vi "example.vi"() -> ()   [LabVIEW 2019]
uses:
  d822b4ab-b711-45da-a8f1-ab7e2b244829.vi
  netCDFModule.py path constant.vi
panel:
  out "return value":dbl[][][][](array[numeric])
  in  "variable key":string
  in  "dimension key":string
  out "dimension":string
  in  "metadata key":string
  in  "file path":path
  out "error out":errorcluster
  out "metadata":string
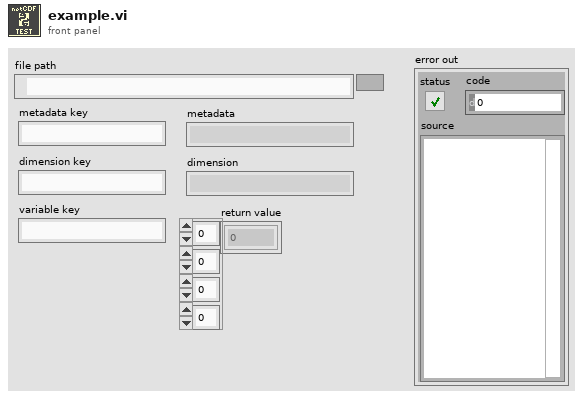
[diagram p1: front panel]
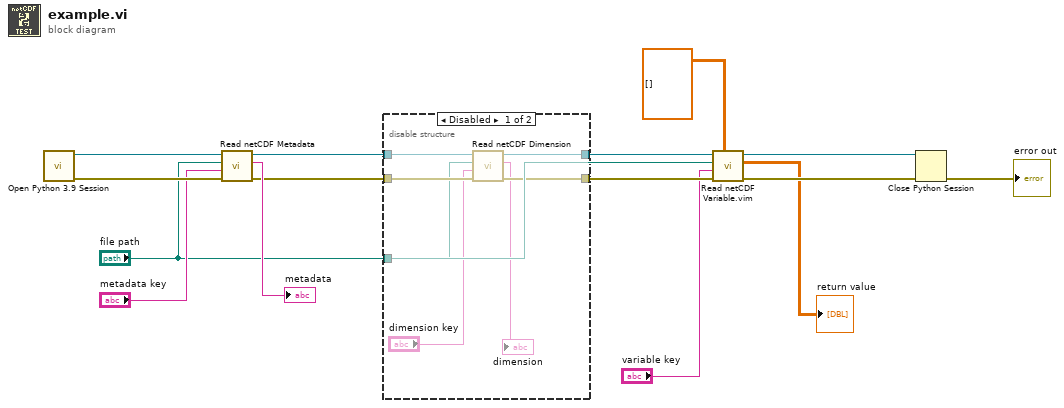
[diagram p0: block diagram]
diagram:
  n1 = call "Open Python 3.9 Session.vi"() -> ("error out"=w15:errorcluster, "Refnum out"=w12:refnum<k35>)  [unwired: 10 in]
  n2 = call "Read netCDF Metadata.vi"("error in (no error)"=w15, "key"="metadata key", "file path"="file path", "Refnum in"=w12) -> ("error out"=w9:errorcluster, "Value"=→"metadata":string, "Refnum out"=w10:refnum<k35>)  [unwired: 5 in]
  n3 = disable-structure shown="Disabled" {
    disable-tunnel: w10 -> [w22 w23]
    disable-tunnel: w9 -> [w21 w24]
    disable-tunnel: "file path" -> [w20 _]
    disable-tunnel: [w19 w23] -> w5
    disable-tunnel: [w18 w24] -> w4
    frame Disabled {
      n4 = call "Read netCDF Dimension.vi"("error in (no error)"=w21, "key"="dimension key", "file path"=w20, "Refnum in"=w22) -> ("error out"=w18:errorcluster, "Dimension"=→"dimension":string, "Refnum out"=w19:refnum<k35>)  [unwired: 5 in]
    }
    frame Enabled {
    }
  }
  n5 = call "Read netCDF Variable.vim"("return type"=dbl[][][][] [], "error in (no error)"=w4, "key"="variable key", "file path"="file path", "Refnum in"=w5) -> ("error out"=w7:errorcluster, "return value"=→"return value":dbl[][][][], "Refnum out"=w8:refnum<k35>)  [unwired: 4 in]
  n6 = Close Python Session(session in=w8, error in=w7) -> (11:→"error out":errorcluster)
